vi "onExecuteJob.vi"(8 "error in (no error)":errorcluster, 10 "stdin":string, 11 "Job in":refnum<class "Job.lvclass">) -> (0 "error out":errorcluster, 1 "exception":i32, 2 "stdout":string, 3 "Job out":refnum<class "Job.lvclass">)   [LabVIEW 2013, in "openCronJob.lvlib" / "Job.lvclass"]
uses:
  Job.lvclass
panel:
  # "RUNNING A JOB"
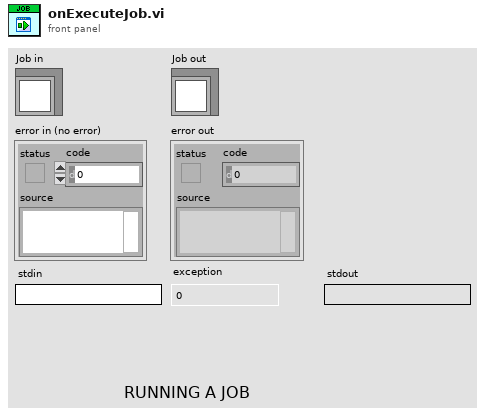
[diagram p1: front panel]
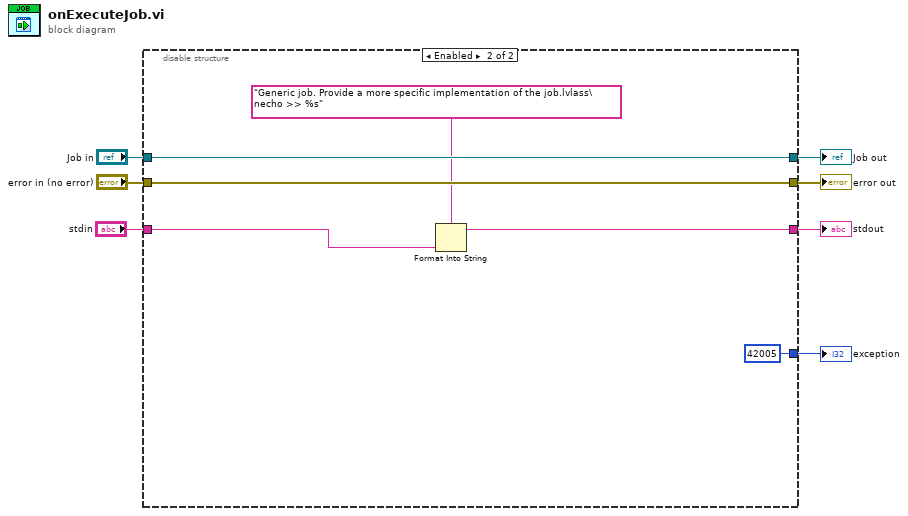
[diagram p0: block diagram]
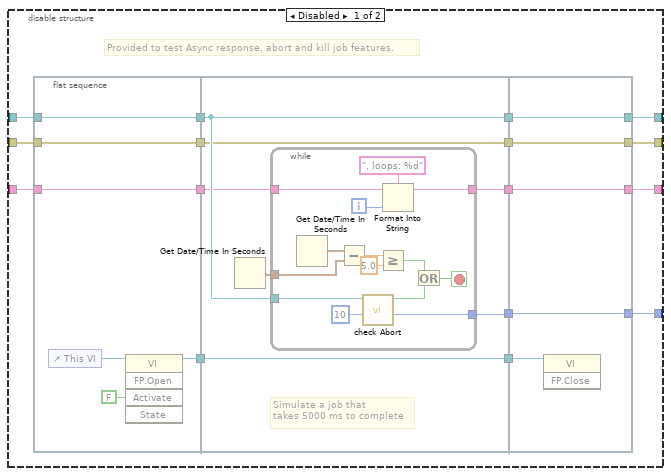
[diagram p2: hidden frame]
diagram:
  n1 = disable-structure shown="Enabled" {
    disable-tunnel: "Job in" -> [w18 w61]
    disable-tunnel: [w21 w61] -> w6
    disable-tunnel: [w17 w60] -> w5
    disable-tunnel: "error in (no error)" -> [w14 w60]
    disable-tunnel: [w13 42005 ("exception")] -> w3
    disable-tunnel: [w11 w58] -> w2
    disable-tunnel: "stdin" -> [w8 w59]
    frame Disabled {
      # "Provided to test Async response, abort and kill job features."
      n2 = flat-sequence {
        tunnel: [w28] -> w22
        tunnel: [w26] -> w19
        tunnel: w18 -> [w26]
        tunnel: [w25] -> w15
        tunnel: w14 -> [w25]
        tunnel: [w24] -> w9
        tunnel: w8 -> [w24]
        tunnel: [w36] -> w23
        tunnel: w22 -> [w36]
        tunnel: [w35] -> w20
        tunnel: w19 -> [w35]
        tunnel: [w34] -> w16
        tunnel: w15 -> [w34]
        tunnel: [w33] -> w12
        tunnel: [w30] -> w10
        tunnel: w9 -> [w31]
        tunnel: w23 -> [w55]
        tunnel: [w54] -> w21
        tunnel: w20 -> [w54]
        tunnel: [w53] -> w17
        tunnel: w16 -> [w53]
        tunnel: [w52] -> w13
        tunnel: w12 -> [w52]
        tunnel: [w51] -> w11
        tunnel: w10 -> [w51]
        frame #0 {
          n3 = control-ref of="This VI"() -> (w29:refnum<vi>)
          n4 = invoke class="VI" method="FP.Open"(reference=w29, "Activate"=FALSE ("Activate?")) -> (reference out=w28:refnum<vi>)  [unwired: 3 in, 4 out]
        }
        frame #1 {
          # "Simulate a job that\ntakes 5000 ms to complete"
          n5 = Get Date/Time In Seconds() -> (seconds since 1Jan1904=w32:timestamp)
          n6 = while {
            tunnel: w35 -> [w50]
            tunnel: [w48] -> w33
            tunnel: w32 -> [w47]
            tunnel: w31 -> [w39]
            tunnel: [w38] -> w30
            i -> [w40]
            stop <- w42 stop-if-true
            n7 = Get Date/Time In Seconds() -> (seconds since 1Jan1904=w41:timestamp)
            n8 = Subtract(x=w41, y=w47) -> (x-y=w46:dbl)
            n9 = call "check Abort.vi"("timeout (0 ms)"=10 ("timeout in ms (-1)"), "Job in"=w50) -> ("exception"=w48:i32, "Abort"=w43:bool)  [unwired: 8 in]
            n10 = Greater Or Equal?(x=w46, y=5.0) -> (x >= y?=w44:bool)
            n11 = Format Into String(format string=", loops: %d", initial string=w39, w40) -> (resulting string=w38:string)  [unwired: 1 in, 1 out]
            n12 = Or(x=w44, y=w43) -> (x .or. y?=w42:bool)
          }
        }
        frame #2 {
          n13 = invoke class="VI" method="FP.Close"(reference=w55) -> ()  [unwired: 2 in, 3 out]
        }
      }
    }
    frame Enabled {
      n14 = Format Into String(format string="Generic job. Provide a more specific implementation of the job.lvlass\necho >> %s", w59) -> (resulting string=w58:string)  [unwired: 2 in, 1 out]
    }
  }
  "error out" <- w5
  "Job out" <- w6
  "exception" <- w3
  "stdout" <- w2
